vi "Wait (with error).vi"(8 "error in (no error)":errorcluster, 10 "milliseconds to wait":u32) -> (0 "error out":errorcluster, 2 "time":timestamp)   [LabVIEW 2016]
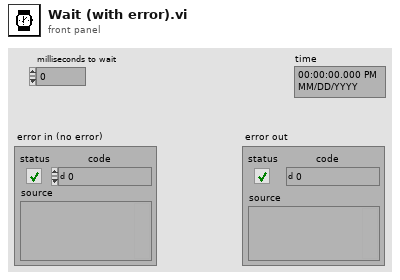
[diagram p1: front panel]
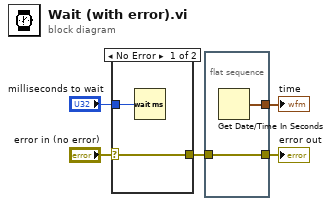
[diagram p0: block diagram]
diagram:
  n1 = case shown="No Error" "error in (no error)" {
    selector: "error in (no error)" -> [w6 w8]
    tunnel: "milliseconds to wait" -> [w7 _]
    tunnel: [w6 w8] -> w3
    frame No Error {
      n2 = Wait (ms)(milliseconds to wait=w7) -> ()  [unwired: 1 out]
    }
    frame Error {
    }
  }
  n3 = flat-sequence {
    tunnel: w3 -> [w10]
    tunnel: [w10] -> w2
    tunnel: [w9] -> w1
    frame #0 {
      n4 = Get Date/Time In Seconds() -> (seconds since 1Jan1904=w9:timestamp)
    }
  }
  "error out" <- w2
  "time" <- w1
